vi "Write.vi"(8 "error in (no error)":errorcluster, 10 "Message":string, 11 "Wifi in":refnum<class "Wifi.lvclass">) -> (0 "error out":errorcluster, 3 "Wifi out":refnum<class "Wifi.lvclass">)   [LabVIEW 2021, in "Wifi.lvclass"]
uses:
  Wifi.lvclass
  Wifi.lvclass/Wifi.ctl
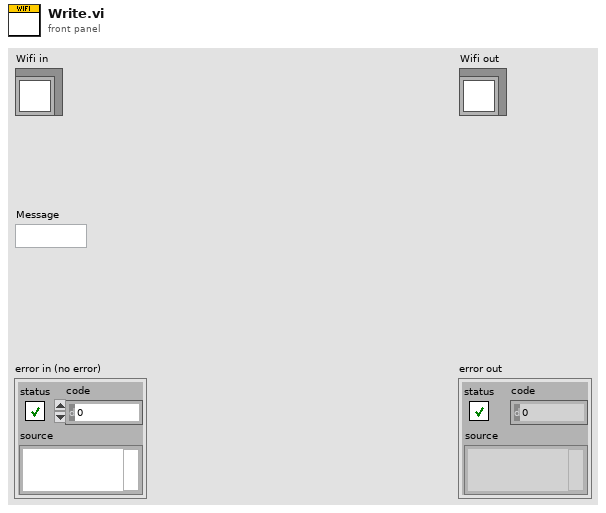
[diagram p1: front panel]
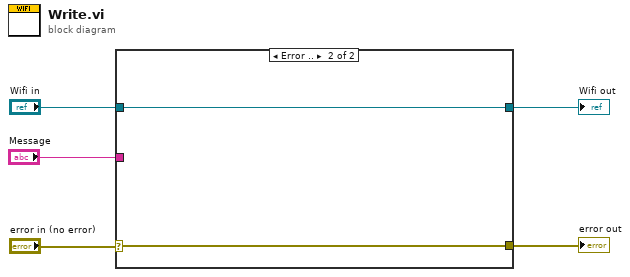
[diagram p0: block diagram]
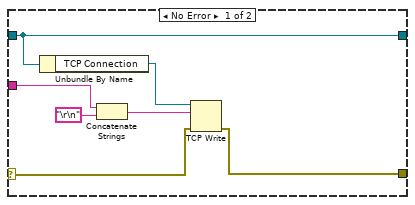
[diagram p2: hidden frame]
diagram:
  n1 = case shown="Error .." "error in (no error)" {
    selector: "error in (no error)" -> [w11 w14]
    tunnel: [w10 w14] -> w4
    tunnel: "Message" -> [w8 _]
    tunnel: "Wifi in" -> [w6 w13]
    tunnel: [w6 w13] -> w1
    frame No Error {
      n2 = Unbundle By Name(w6) -> ("TCP Connection"=w7:refnum<k5>)
      n3 = Concatenate Strings(w8, "\r\n") -> (w12:string)
      n4 = TCP Write(connection ID=w7, data in=w12, error in (no error)=w11) -> (error out=w10:errorcluster)  [unwired: 1 in, 2 out]
    }
    frame Error {
    }
  }
  "error out" <- w4
  "Wifi out" <- w1
